vi "Untitled 4.vi"() -> ()   [LabVIEW 2023]
uses:
  <vilib>/Rock Robotics/WPI/ThirdParty/JAS_Junk/TrajLib/TypeDef/SWERVE_DRIVE_KINEMATICS.ctl
  <vilib>/Analysis/Matrix/Datatypes/RealMatrix.ctl
  <vilib>/Rock Robotics/WPI/ThirdParty/JAS_Junk/TrajLib/TypeDef/TRANSLATION2D.ctl
  <vilib>/Rock Robotics/WPI/ThirdParty/JAS_Junk/TrajLib/TypeDef/SWERVE_DRIVE_MODULE_STATE.ctl
  <vilib>/Rock Robotics/WPI/ThirdParty/JAS_Junk/TrajLib/TypeDef/ROTATION2D.ctl
  <vilib>/Analysis/Matrix/NI_Matrix.lvlib
  <vilib>/Analysis/Matrix/Comparison/Equal/Equal - RM,RM.vi
  <vilib>/Rock Robotics/WPI/ThirdParty/JAS_Junk/TrajLib/Trajectory_Library.lvlib
panel:
  in  "SWERVE_DRIVE_KINEMATICS 3":T1 {"SavedModuleStates"."Angle"."SIN" format="%13.4f"; "SavedModuleStates"."Angle"."COS" format="%13.4f"; "SavedModuleStates"."Angle"."VALUE" format="%13.4f"; "PrevCoR"."Y" format="%14.3f"; "PrevCoR"."X" format="%14.3f"; "Modules"."Y" format="%14.3f"; "Modules"."X" format="%14.3f"}
  in  "SWERVE_DRIVE_KINEMATICS 2":T1 {"SavedModuleStates"."Angle"."SIN" format="%13.4f"; "SavedModuleStates"."Angle"."COS" format="%13.4f"; "SavedModuleStates"."Angle"."VALUE" format="%13.4f"; "PrevCoR"."Y" format="%14.3f"; "PrevCoR"."X" format="%14.3f"; "Modules"."Y" format="%14.3f"; "Modules"."X" format="%14.3f"}
  out "Variant":variant
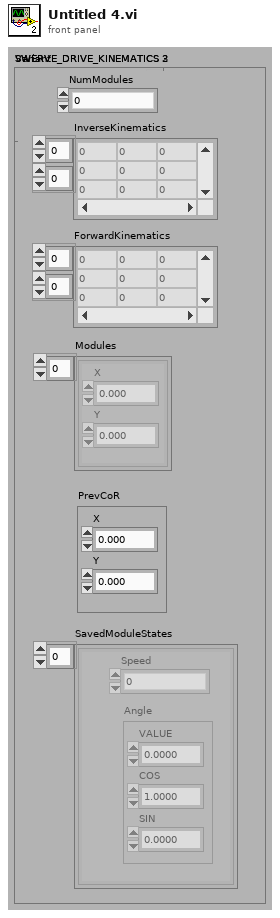
[diagram p1: front panel]
types:
  T1 = typedef "Trajectory_Library.lvlib/SWERVE_DRIVE_KINEMATICS.ctl" = cluster{"NumModules":i32, "InverseKinematics":T2, "ForwardKinematics":T2, "Modules":T3[], "PrevCoR":T3, "SavedModuleStates":T4[]}
  T2 = typedef "NI_Matrix.lvlib/RealMatrix.ctl" = dbl[][]
  T3 = typedef "Trajectory_Library.lvlib/TRANSLATION2D.ctl" = cluster{"X":dbl, "Y":dbl}
  T4 = typedef "Trajectory_Library.lvlib/SWERVE_DRIVE_MODULE_STATE.ctl" = cluster{"Speed":dbl, "Angle":T5}
  T5 = typedef "Trajectory_Library.lvlib/ROTATION2D.ctl" = cluster{"VALUE":dbl, "COS":dbl, "SIN":dbl}
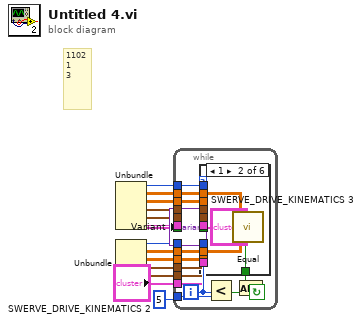
[diagram p0: block diagram]
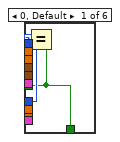
[diagram p2: hidden frame]
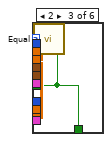
[diagram p3: hidden frame]
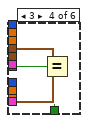
[diagram p4: hidden frame]
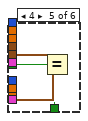
[diagram p5: hidden frame]
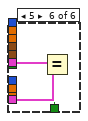
[diagram p6: hidden frame]
diagram:
  # "1102\n1\n3"
  n1 = Unbundle("SWERVE_DRIVE_KINEMATICS 3") -> ("NumModules"=w6:i32, "InverseKinematics"=w5:T2, "ForwardKinematics"=w4:T2, "Modules"=w3:T3[], "PrevCoR"=w2:T3, "SavedModuleStates"=w1:T4[])
  n2 = Unbundle("SWERVE_DRIVE_KINEMATICS 2") -> ("NumModules"=w12:i32, "InverseKinematics"=w11:T2, "ForwardKinematics"=w10:T2, "Modules"=w9:T3[], "PrevCoR"=w8:T3, "SavedModuleStates"=w7:T4[])
  n3 = while {
    tunnel: 5 -> [w32]
    tunnel: [w29] -> w13
    tunnel: w12 -> [w28]
    tunnel: w11 -> [w27]
    tunnel: w10 -> [w26]
    tunnel: w9 -> [w25]
    tunnel: w8 -> [w24]
    tunnel: w7 -> [w23]
    tunnel: w6 -> [w22]
    tunnel: w5 -> [w21]
    tunnel: w4 -> [w20]
    tunnel: w3 -> [w19]
    tunnel: w2 -> [w18]
    tunnel: w1 -> [w17]
    i -> [w33]
    stop <- w34 continue-if-true
    n4 = case shown="1" w33 {
      tunnel: [w35 w38 w41 w44 w47 w50] -> w30
      tunnel: [w35 w38 w41 w44 w47 w50] -> w29
      tunnel: w28 -> [w36 _ _ _ _ _]
      tunnel: w27 -> [_ w39 _ _ _ _]
      tunnel: w26 -> [_ _ w42 _ _ _]
      tunnel: w25 -> [_ _ _ w45 _ _]
      tunnel: w24 -> [_ _ _ _ w48 _]
      tunnel: w23 -> [_ _ _ _ _ w51]
      tunnel: w22 -> [w37 _ _ _ _ _]
      tunnel: w21 -> [_ w40 _ _ _ _]
      tunnel: w20 -> [_ _ w43 _ _ _]
      tunnel: w19 -> [_ _ _ w46 _ _]
      tunnel: w18 -> [_ _ _ _ w49 _]
      tunnel: w17 -> [_ _ _ _ _ w52]
      frame 0, Default {
        n5 = Equal?(x=w37, y=w36) -> (x = y?=w35:bool)
      }
      frame 1 {
        n6 = call-poly <vilib>:"Equal.vi"("Real Matrix B"=w39, "Real Matrix A"=w40) -> ("A = B?"=w38:bool)
      }
      frame 2 {
        n7 = call-poly <vilib>:"Equal.vi"("Real Matrix B"=w42, "Real Matrix A"=w43) -> ("A = B?"=w41:bool)
      }
      frame 3 {
        n8 = Equal?(x=w46, y=w45) -> (x = y?=w44:bool)
      }
      frame 4 {
        n9 = Equal?(x=w49, y=w48) -> (x = y?=w47:bool)
      }
      frame 5 {
        n10 = Equal?(x=w52, y=w51) -> (x = y?=w50:bool)
      }
    }
    n11 = Less?(x=w33, y=w32) -> (x < y?=w31:bool)
    n12 = And(x=w30, y=w31) -> (x .and. y?=w34:bool)
  }
  "Variant" <- w13
